vi "translate_settings.vi"(6 "error in":errorcluster, 9 "GenericClock in":refnum<class "ClockDL100201DAQmx.lvclass">) -> (0 "error out":errorcluster, 3 "GenericClock out":refnum<class "ClockDL100201DAQmx.lvclass">)   [LabVIEW 2010, in "ClockDL100201DAQmx.lvclass"]
uses:
  ClockDL100201DAQmx.lvclass
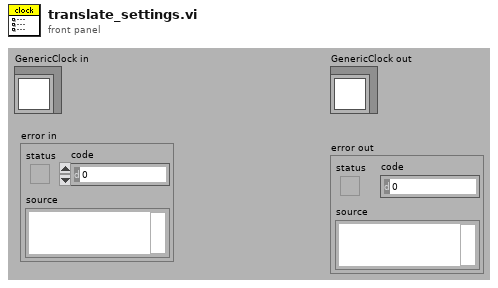
[diagram p1: front panel]
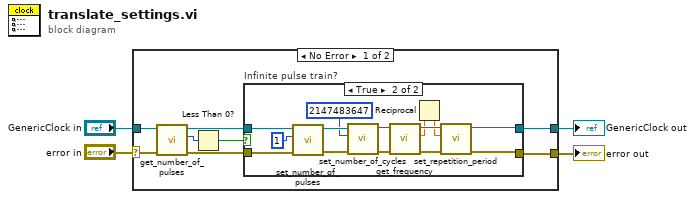
[diagram p0: block diagram]
diagram:
  n1 = case shown="No Error" "error in" {
    selector: "error in" -> [w11 w29]
    tunnel: "GenericClock in" -> [w12 w30]
    tunnel: [w7 w30] -> w4
    tunnel: [w5 w29] -> w1
    frame No Error {
      n2 = call-dynamic "get_number_of_pulses.vi"("error in (no error)"=w11, "GenericClock.lvclass in"=w12) -> ("error out"=w6:errorcluster, "number of pulses"=w10:i64, "GenericClock.lvclass out"=w8:refnum<class "ClockDL100201DAQmx.lvclass">)  [unwired: 7 in]
      n3 = Less Than 0?(x=w10) -> (x < 0?=w9:bool)
      n4 = case "Infinite pulse train?" shown="True" w9 {
        tunnel: w8 -> [w14 w27]
        tunnel: [w14 w16] -> w7
        tunnel: [w13 w15] -> w5
        tunnel: w6 -> [w13 w28]
        frame False {
          # "Not an infinite pulse train. Just pass the data trough!"
        }
        frame True {
          n5 = call-dynamic "set_number_of_pulses.vi"("error in (no error)"=w28, "number of pulses"=i64 1, "GenericClock.lvclass in"=w27) -> ("error out"=w24:errorcluster, "GenericClock.lvclass out"=w25:refnum<class "ClockDL100201DAQmx.lvclass">)  [unwired: 7 in]
          n6 = call-dynamic "set_number_of_cycles.vi"("error in (no error)"=w24, "number of cycles"=i64 2147483647, "GenericClock.lvclass in"=w25) -> ("error out"=w21:errorcluster, "GenericClock.lvclass out"=w22:refnum<class "ClockDL100201DAQmx.lvclass">)  [unwired: 7 in]
          n7 = call-dynamic "get_frequency.vi"("error in (no error)"=w21, "GenericClock.lvclass in"=w22) -> ("error out"=w19:errorcluster, "frequency"=w18:dbl[unit], "GenericClock.lvclass out"=w20:refnum<class "ClockDL100201DAQmx.lvclass">)  [unwired: 7 in]
          n8 = Reciprocal(x=w18) -> (1/x=w17:dbl[unit])
          n9 = call-dynamic "set_repetition_period.vi"("error in (no error)"=w19, "repetition period"=w17, "GenericClock.lvclass in"=w20) -> ("error out"=w15:errorcluster, "GenericClock.lvclass out"=w16:refnum<class "ClockDL100201DAQmx.lvclass">)  [unwired: 7 in]
        }
      }
    }
    frame Error {
    }
  }
  "error out" <- w1
  "GenericClock out" <- w4
